vi "return2.vi"(9 "Colors and Directions":enum16{"Zero", "Right", "Front", "Left"}[](array[ring])=[enum."Zero", enum."Zero", enum."Zero", enum."Zero", enum."Zero", enum."Zero"], 11 "NXT/EV3":T1) -> (1 "Colors and Directions 2":enum16{"Zero", "Right", "Front", "Left"}[](array[ring])=[enum."Zero", enum."Zero", enum."Zero", enum."Zero", enum."Zero", enum."Zero"], 3 "NXT/EV3 2":T1)   [LabVIEW 2016]
uses:
  <vilib>/NXT/Subs/LVHSConnector.ctl
  <vilib>/NXT/LegoClasses/BrickReference/BrickReference.lvclass
  <vilib>/NXT/Subs/ColorSensorColors.ctl
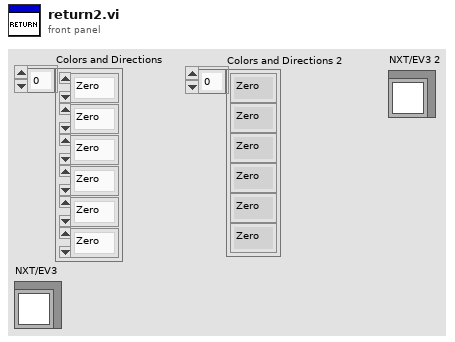
[diagram p1: front panel]
types:
  T1 = typedef "LVHSConnector.ctl" = refnum<class "BrickReference.lvclass">
  T2 = typedef "ColorSensorColors.ctl" = enum16{"No Color", "Black", "Blue", "Green", "Yellow", "Red", "White", "Brown"}
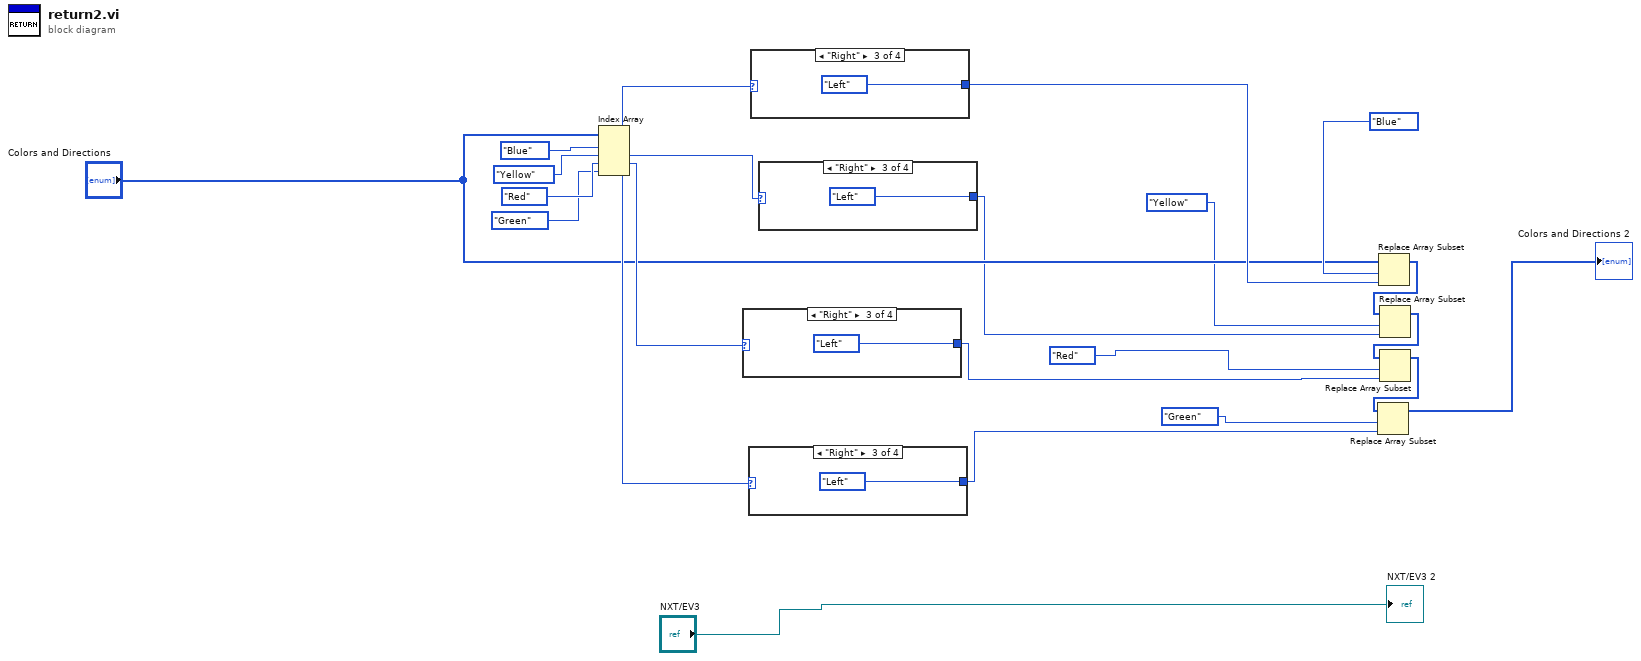
[diagram p0: block diagram]
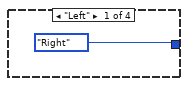
[diagram p2: hidden frame]
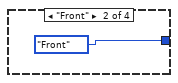
[diagram p3: hidden frame]
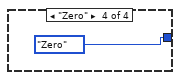
[diagram p4: hidden frame]
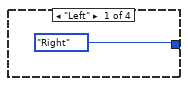
[diagram p5: hidden frame]
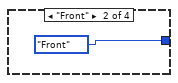
[diagram p6: hidden frame]
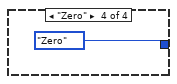
[diagram p7: hidden frame]
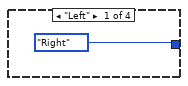
[diagram p8: hidden frame]
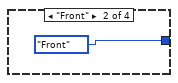
[diagram p9: hidden frame]
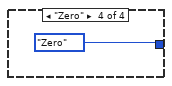
[diagram p10: hidden frame]
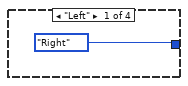
[diagram p11: hidden frame]
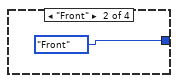
[diagram p12: hidden frame]
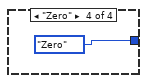
[diagram p13: hidden frame]
diagram:
  n1 = Index Array(array="Colors and Directions", index #1=ColorSensorColors."Blue" ("Detected Color"), index #2=ColorSensorColors."Yellow" ("Detected Color"), index #3=ColorSensorColors."Red" ("Detected Color"), index #4=ColorSensorColors."Green" ("Detected Color")) -> (element #1=w17:enum16{"Zero", "Right", "Front", "Left"}, element #2=w15:enum16{"Zero", "Right", "Front", "Left"}, element #3=w14:enum16{"Zero", "Right", "Front", "Left"}, element #4=w13:enum16{"Zero", "Right", "Front", "Left"})
  n2 = case shown="\"Right\"" w14 {
    tunnel: [enum16{"Zero", "Right", "Front", "Left"}."Right" ("Direction") enum16{"Zero", "Right", "Front", "Left"}."Front" ("Direction") enum16{"Zero", "Right", "Front", "Left"}."Left" ("Direction") enum16{"Zero", "Right", "Front", "Left"}."Zero" ("Direction")] -> w3
    frame "Left" {
    }
    frame "Front" {
    }
    frame "Right" {
    }
    frame "Zero" {
    }
  }
  n3 = case shown="\"Right\"" w13 {
    tunnel: [enum16{"Zero", "Right", "Front", "Left"}."Right" ("Direction") enum16{"Zero", "Right", "Front", "Left"}."Front" ("Direction") enum16{"Zero", "Right", "Front", "Left"}."Left" ("Direction") enum16{"Zero", "Right", "Front", "Left"}."Zero" ("Direction")] -> w1
    frame "Left" {
    }
    frame "Front" {
    }
    frame "Right" {
    }
    frame "Zero" {
    }
  }
  n4 = case shown="\"Right\"" w17 {
    tunnel: [enum16{"Zero", "Right", "Front", "Left"}."Right" ("Direction") enum16{"Zero", "Right", "Front", "Left"}."Front" ("Direction") enum16{"Zero", "Right", "Front", "Left"}."Left" ("Direction") enum16{"Zero", "Right", "Front", "Left"}."Zero" ("Direction")] -> w16
    frame "Left" {
    }
    frame "Front" {
    }
    frame "Right" {
    }
    frame "Zero" {
    }
  }
  n5 = case shown="\"Right\"" w15 {
    tunnel: [enum16{"Zero", "Right", "Front", "Left"}."Right" ("Direction") enum16{"Zero", "Right", "Front", "Left"}."Front" ("Direction") enum16{"Zero", "Right", "Front", "Left"}."Left" ("Direction") enum16{"Zero", "Right", "Front", "Left"}."Zero" ("Direction")] -> w5
    frame "Left" {
    }
    frame "Front" {
    }
    frame "Right" {
    }
    frame "Zero" {
    }
  }
  n6 = Replace Array Subset(array="Colors and Directions", new element=w16, index=ColorSensorColors."Blue" ("Detected Color")) -> (w10:enum16{"Zero", "Right", "Front", "Left"}[])
  n7 = Replace Array Subset(array=w10, new element=w5, index=ColorSensorColors."Yellow" ("Detected Color")) -> (w9:enum16{"Zero", "Right", "Front", "Left"}[])
  n8 = Replace Array Subset(array=w9, new element=w3, index=ColorSensorColors."Red" ("Detected Color")) -> (w8:enum16{"Zero", "Right", "Front", "Left"}[])
  n9 = Replace Array Subset(array=w8, new element=w1, index=ColorSensorColors."Green" ("Detected Color")) -> (→"Colors and Directions 2":enum16{"Zero", "Right", "Front", "Left"}[])
  "NXT/EV3 2" <- "NXT/EV3"
